vi "switchPressure_topLvl.vi"(5 "which manipulator":T1(ring), 7 "Slide Refnum":refnum<vi>, 8 "error in":errorcluster, 10 "pressure setting":T2, 11 "Pressure box control in":T3={"Pressure box COM"="", "pressure box type"=enum."Neuromatics", "High pos pressure (mBar)"=200.0, "Low pos pressure (mBar)"=80.0, "Vacuum pressure (mBar)"=-40.0, "calibration"=enum."PA_vacPump"}) -> (0 "error out":errorcluster, 3 "Pressure box control out":T3={"Pressure box COM"="", "pressure box type"=enum."Neuromatics", "High pos pressure (mBar)"=200.0, "Low pos pressure (mBar)"=80.0, "Vacuum pressure (mBar)"=-40.0, "calibration"=enum."PA_vacPump"})   [LabVIEW 2015]
uses:
  controls/proportionAir_cmds.ctl
  controls/arduino_pressure_setting.ctl
  controls/pressure_box_type.ctl
  controls/pressure_box_control.ctl
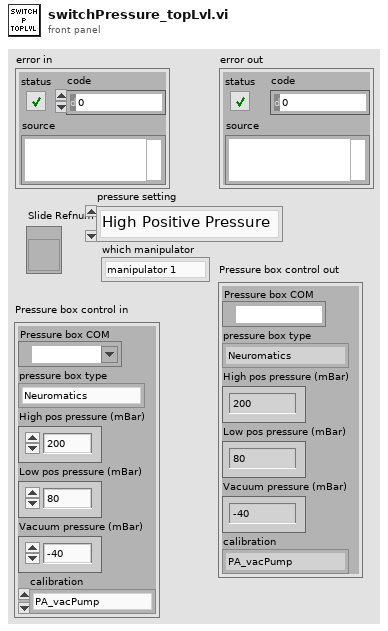
[diagram p1: front panel]
types:
  T1 = enum16{"manipulator 1", "manipulator 2", "manipulator 3", "manipulator 4"}
  T2 = typedef "arduino_pressure_setting.ctl" = enum16{"High Positive Pressure", "Low Positive Pressure", "Atmospheric Pressure", "Low Vacuum", "High Vacuum", "Break In", "Puff"}
  T3 = typedef "pressure_box_control.ctl" = cluster{"Pressure box COM":refnum<visa-resource-name>, "pressure box type":T4, "High pos pressure (mBar)":dbl, "Low pos pressure (mBar)":dbl, "Vacuum pressure (mBar)":dbl, "calibration":enum16{"PA_vacPump", "PA_venturi", "Neuromatics", "ilyaRig", "mightenRig"}}
  T4 = typedef "pressure_box_type.ctl" = enum16{"Neuromatics", "ProportionAir", "Demo box", "N-ProportionAir"}
  T5 = enum16{"PA_vacPump", "PA_venturi", "Neuromatics", "ilyaRig", "mightenRig"}
  T6 = typedef "proportionAir_cmds.ctl" = enum16{"Set P", "Switch to Atm", "Switch to Regulator", "Pulse", "WC"}
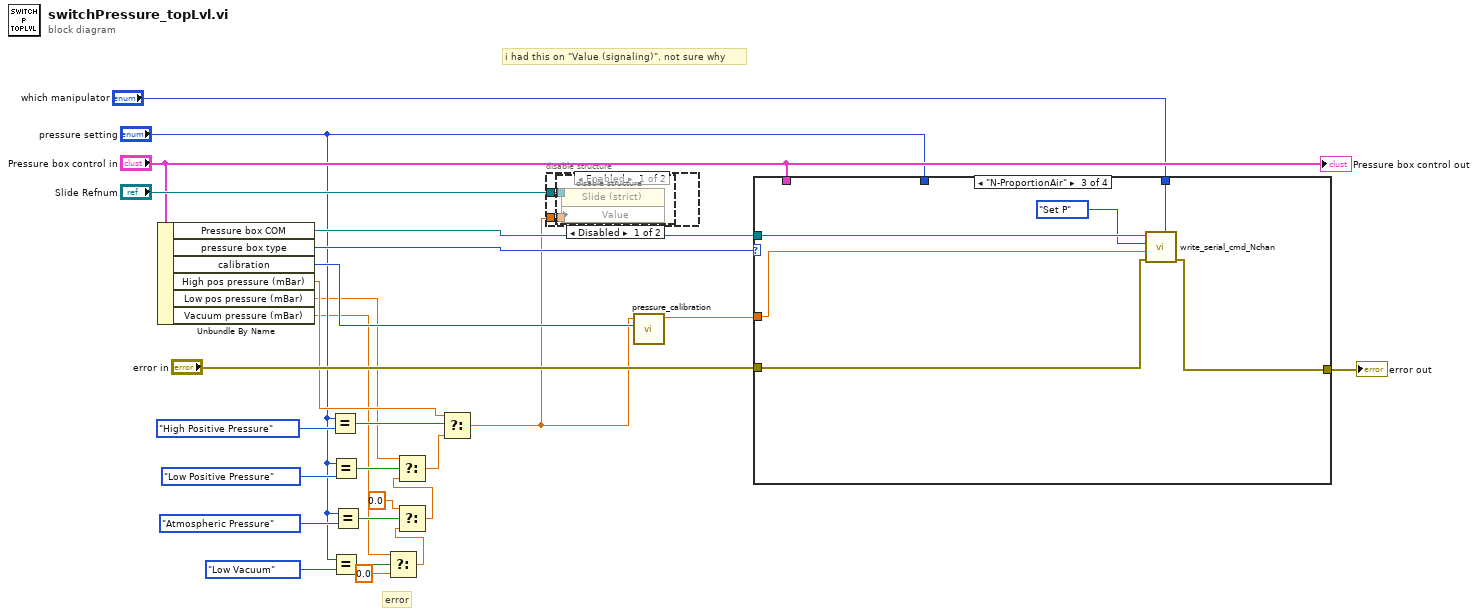
[diagram p0: block diagram]
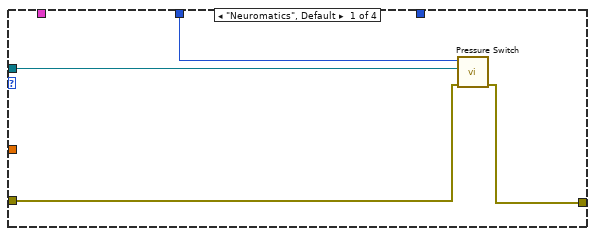
[diagram p4: hidden frame]
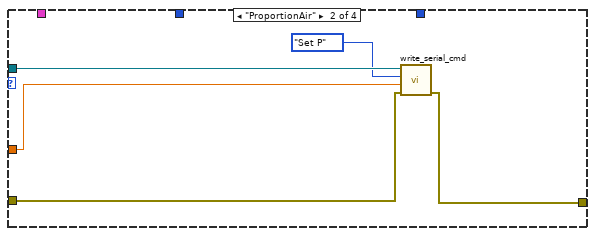
[diagram p5: hidden frame]
diagram:
  # "error"
  # "i had this on \"Value (signaling)\". not sure why"
  n1 = Unbundle By Name("Pressure box control in") -> ("Pressure box COM"=w26:refnum<visa-resource-name>, "pressure box type"=w27:T4, "calibration"=w22:T5, "High pos pressure (mBar)"=w17:dbl, "Low pos pressure (mBar)"=w4:dbl, "Vacuum pressure (mBar)"=w3:dbl)
  n2 = Equal?(x="pressure setting", y=arduino_pressure_setting."High Positive Pressure" ("pressure setting")) -> (x = y?=w18:bool)
  n3 = Equal?(x="pressure setting", y=arduino_pressure_setting."Low Positive Pressure" ("pressure setting")) -> (x = y?=w14:bool)
  n4 = Equal?(x="pressure setting", y=arduino_pressure_setting."Low Vacuum" ("pressure setting")) -> (x = y?=w8:bool)
  n5 = Equal?(x="pressure setting", y=arduino_pressure_setting."Atmospheric Pressure" ("pressure setting")) -> (x = y?=w12:bool)
  n6 = Select(t=w3, s=w8, f=0.0) -> (s? t:f=w9:dbl)
  n7 = Select(t=0.0, s=w12, f=w9) -> (s? t:f=w13:dbl)
  n8 = Select(t=w4, s=w14, f=w13) -> (s? t:f=w16:dbl)
  n9 = Select(t=w17, s=w18, f=w16) -> (s? t:f=w5:dbl)
  n10 = disable-structure shown="Enabled" {
    disable-tunnel: "Slide Refnum" -> [w29 _]
    disable-tunnel: w5 -> [w28 _]
    frame Enabled {
      n11 = disable-structure shown="Disabled" {
        disable-tunnel: w29 -> [w31 _]
        disable-tunnel: w28 -> [w30 _]
        frame Disabled {
          n12 = property class="Slide (strict)"(reference=w31, "Value"=w30) -> ()  [unwired: 1 in, 2 out]
        }
        frame Enabled {
        }
      }
    }
    frame Disabled {
    }
  }
  n13 = call "pressure_calibration.vi"("calibration"=w22, "cmd pressure (mBar)"=w5) -> ("pressure out (mbar)"=w23:dbl)  [unwired: 9 in]
  n14 = case shown="\"N-ProportionAir\"" w27 {
    tunnel: w26 -> [w34 w40 w46 _]
    tunnel: "error in" -> [w32 w39 w45 w47]
    tunnel: w23 -> [_ w36 w42 _]
    tunnel: [w35 w38 w44 w47] -> w24
    tunnel: "pressure setting" -> [w33 _ _ _]
    tunnel: "Pressure box control in" -> [_ _ _ _]
    tunnel: "which manipulator" -> [_ _ w41 _]
    frame "Neuromatics", Default {
      n15 = call "Pressure Switch.vi"("error in"=w32, "Pressure Box COM"=w34, "arduino pressure setting"=w33) -> ("error out"=w35:errorcluster)  [unwired: 7 in, 1 out]
    }
    frame "ProportionAir" {
      n16 = call "write_serial_cmd.vi"("error in"=w39, "pressure set (mBar)"=w36, "pressure command"=proportionAir_cmds."Set P", "Pressure Box COM"=w40) -> ("error out"=w38:errorcluster)  [unwired: 6 in, 1 out]
    }
    frame "N-ProportionAir" {
      n17 = call "write_serial_cmd_Nchan.vi"("which manipulator"=w41, "error in"=w45, "arg 1"=w42, "pressure command"=proportionAir_cmds."Set P", "Pressure Box COM"=w46) -> ("error out"=w44:errorcluster)  [unwired: 5 in, 1 out]
    }
    frame "Demo box" {
    }
  }
  "error out" <- w24
  "Pressure box control out" <- "Pressure box control in"
